vi "getObservers.vi"(8 "error in (no error)":errorcluster, 11 "Observable in":refnum<class "Observable.lvclass">) -> (0 "error out":errorcluster, 2 "Observers":refnum<class "Observer.lvclass">[](array[class]), 3 "Observable out":refnum<class "Observable.lvclass">)   [LabVIEW 2017, in "Observable.lvclass"]
uses:
  Observable.lvclass
  Observer/Observer.lvclass
  Observable.lvclass/Observable.ctl
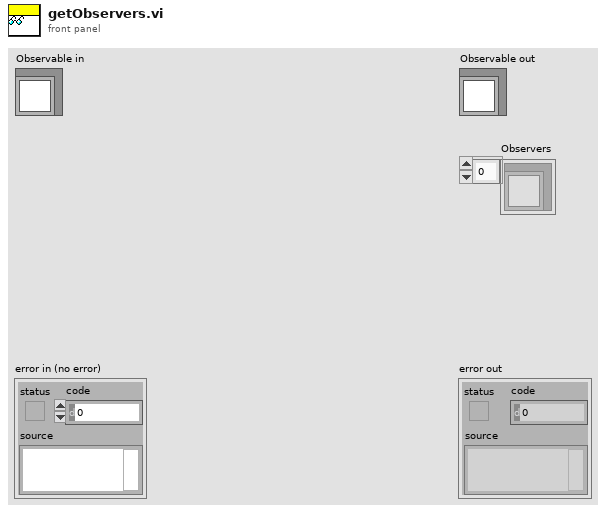
[diagram p1: front panel]
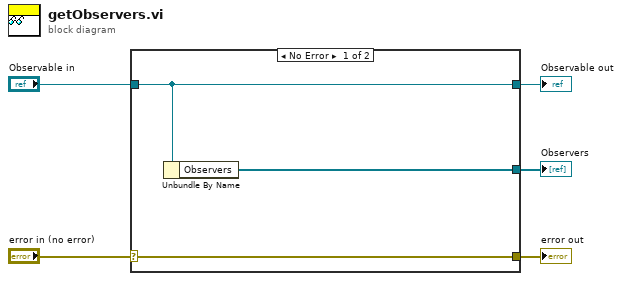
[diagram p0: block diagram]
diagram:
  n1 = case shown="No Error" "error in (no error)" {
    selector: "error in (no error)" -> [w8 w9]
    tunnel: [w8 w9] -> w4
    tunnel: [w7 w10] -> w2
    tunnel: "Observable in" -> [w7 w10]
    tunnel: [w6 _] -> w1
    frame No Error {
      n2 = Unbundle By Name(w7) -> ("Observers"=w6:refnum<class "Observer.lvclass">[])
    }
    frame Error {
    }
  }
  "error out" <- w4
  "Observable out" <- w2
  "Observers" <- w1
